vi "PID.vi"(6 "reinitialize? (F)":bool, 8 "error in (no error)":errorcluster, 9 "process variable":dbl, 10 "setpoint":dbl, 11 "PID in":refnum<class "PID.lvclass">) -> (0 "error out":errorcluster, 2 "output":dbl, 3 "PID out":refnum<class "PID.lvclass">)   [LabVIEW 2024, in "PID.lvlib" / "PID.lvclass"]
uses:
  PID.lvclass
  PID.lvclass/PID.ctl
  <vilib>/addons/control/pid/NI_PID_pid.lvlib
  <vilib>/addons/control/pid/pid.llb/PID (DBL).vi
  <vilib>/addons/control/pid/pid.llb/PID Control Input Filter (DBL).vi
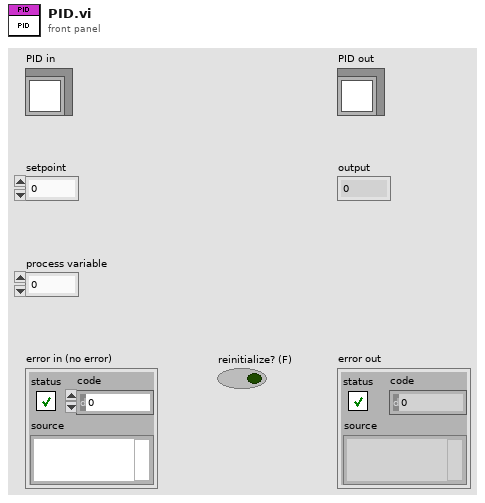
[diagram p1: front panel]
types:
  T1 = cluster{"proportional gain (Kc)":dbl, "integral time (Ti, min)":dbl, "derivative time (Td, min)":dbl}
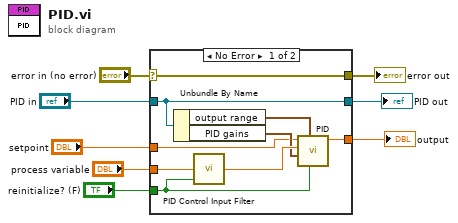
[diagram p0: block diagram]
diagram:
  n1 = case shown="No Error" "error in (no error)" {
    selector: "error in (no error)" -> [w17 w19]
    tunnel: [w17 w19] -> w7
    tunnel: [w15 w18] -> w5
    tunnel: "PID in" -> [w15 w18]
    tunnel: [w12 _] -> w4
    tunnel: "setpoint" -> [w11 _]
    tunnel: "process variable" -> [w10 _]
    tunnel: "reinitialize? (F)" -> [w9 _]
    frame No Error {
      n2 = Unbundle By Name(w15) -> ("output range"=w14:cluster{"output high":dbl, "output low":dbl}, "PID gains"=w13:T1)
      n3 = call-poly <vilib>:"PID Control Input Filter.vi"("reinitialize? (F)"=w9, "input"=w10) -> ("output"=w16:dbl)  [unwired: 3 in]
      n4 = call-poly <vilib>:"PID.vi"("reinitialize? (F)"=w9, "output range"=w14, "PID gains"=w13, "process variable"=w16, "setpoint"=w11) -> ("output"=w12:dbl)  [unwired: 5 in, 1 out]
    }
    frame Error {
    }
  }
  "error out" <- w7
  "PID out" <- w5
  "output" <- w4
